vi "Cancel Observer.vi"(8 "error in (no error)":errorcluster, 11 "CancelableObserver in":refnum<class "CancelableObserver.lvclass">) -> (0 "error out":errorcluster)   [LabVIEW 2011, in "Messenging.lvlib" / "CancelableObserver.lvclass"]
uses:
  CancelableObserver.lvclass
  CancelableObserver.lvclass/CancelableObserver.ctl
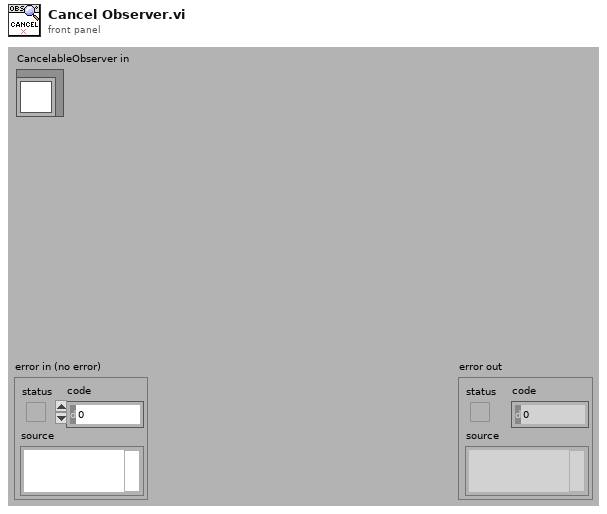
[diagram p1: front panel]
types:
  T1 = typedef "Semaphore RefNum" = refnum<k1>
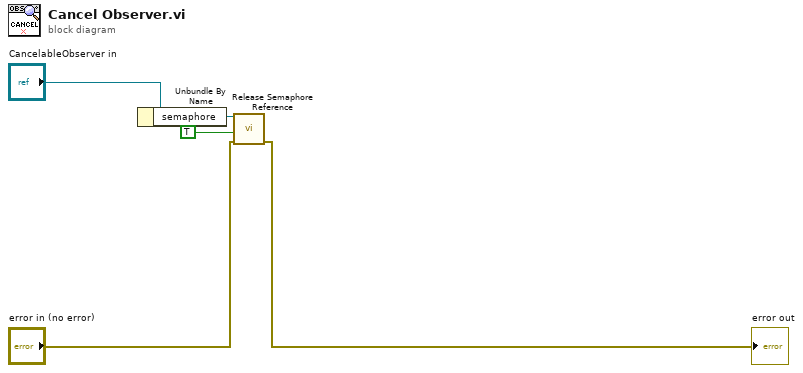
[diagram p0: block diagram]
diagram:
  n1 = Unbundle By Name("CancelableObserver in") -> ("semaphore"=w4:T1)
  n2 = call <vilib>:"Release Semaphore Reference.vi"("error in (no error)"="error in (no error)", "force destroy? (F)"=TRUE, "semaphore"=w4) -> ("error out"=→"error out":errorcluster)  [unwired: 8 out]
